vi "_Open Explorer Window.vi"(8 "error in (no error)":errorcluster, 10 "Select Directory? (F: Open Directory)":bool, 11 "Directory or File":path) -> (0 "error out":errorcluster)   [LabVIEW 2017, in "Smart Open VI Location.lvlib"]
doc: "Open a Windows Explorer window to the specified file's directory and select the file. If the path specifies a directory, then the explorer window is opened to that directory, unless \"Select Directory?\" is true, in which case the explorer window is opened to the parent directory and the specified directory is selected.\n\nAuthored by Shawn Walpole\nsupport@mooregoodideas.com\nwww.mooregoodideas.com\n\nCopyright (c) 2010, Moore Good Ideas, Inc.\n\nAll rights reserved.\n\nRedistribution and use in source and binary forms, with or without modification, are permitted provided that the following conditions are met:\n\n * Redistributions of source code must retain the above copyright notice, this list of conditions and the following disclaimer.\n * Redistributions in binary form must reproduce the above copyright notice, this list of conditions and the following disclaimer in the documentation and/or other materials provided with the distribution.\n * Neither the name of Moore Good Ideas, Inc. nor the names of its contributors may be used to endorse or promote products derived from this software without specific prior written permission.\n\nTHIS SOFTWARE IS PROVIDED BY THE COPYRIGHT HOLDERS AND CONTRIBUTORS \"AS IS\" AND ANY EXPRESS OR IMPLIED WARRANTIES, INCLUDING, BUT NOT LIMITED TO, THE IMPLIED WARRANTIES OF MERCHANTABILITY AND FITNESS FOR A PARTICULAR PURPOSE ARE DISCLAIMED. IN NO EVENT SHALL THE COPYRIGHT OWNER OR CONTRIBUTORS BE LIABLE FOR ANY DIRECT, INDIRECT, INCIDENTAL, SPECIAL, EXEMPLARY, OR CONSEQUENTIAL DAMAGES (INCLUDING, BUT NOT LIMITED TO, PROCUREMENT OF SUBSTITUTE GOODS OR SERVICES; LOSS OF USE, DATA, OR PROFITS; OR BUSINESS INTERRUPTION) HOWEVER CAUSED AND ON ANY THEORY OF LIABILITY, WHETHER IN CONTRACT, STRICT LIABILITY, OR TORT (INCLUDING NEGLIGENCE OR OTHERWISE) ARISING IN ANY WAY OUT OF THE USE OF THIS SOFTWARE, EVEN IF ADVISED OF THE POSSIBILITY OF SUCH DAMAGE."
uses:
  Smart Open VI Location.lvlib
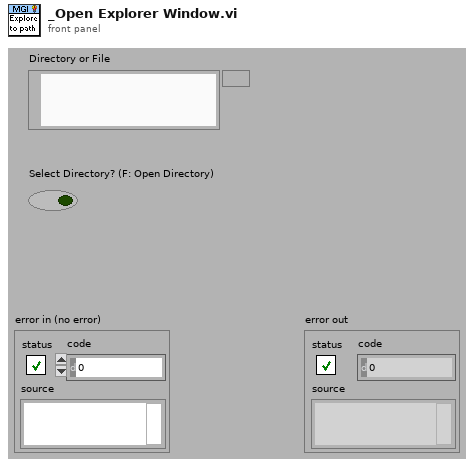
[diagram p1: front panel]
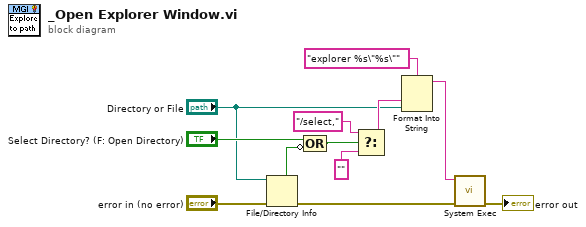
[diagram p0: block diagram]
diagram:
  n1 = File/Directory Info(path="Directory or File", error in="error in (no error)") -> (directory=w9:bool, error out=w7:errorcluster)  [unwired: 5 out]
  n2 = Compound Arithmetic op=OR("Select Directory? (F: Open Directory)", invert w9) -> (w5:bool)
  n3 = Select(t="/select," ("format string"), s=w5, f="") -> (s? t:f=w4:string)
  n4 = Format Into String(format string="explorer %s\"%s\"", w4, "Directory or File") -> (resulting string=w11:string)  [unwired: 2 in, 1 out]
  n5 = call <vilib>:"System Exec.vi"("error in (no error)"=w7, "command line"=w11) -> ("error out"=→"error out":errorcluster)  [unwired: 6 in, 3 out]
